vi "Grabber State Machine.vi"(8 "location of arms":dbl, 9 "grabber control buttons":T1, 10 "Limit Switches":cluster{"guideL":bool, "guideR":bool}, 11 "Laststate":T3) -> (0 "suctioncup":T2, 1 "Pickup Motor":dbl(knob) scale=-1.0..1.0, 3 "Next state":T3)   [LabVIEW 2012]
uses:
  Grabber States.ctl
  <vilib>/Rock Robotics/WPI/Solenoid/WPI_SolenoidValue.ctl
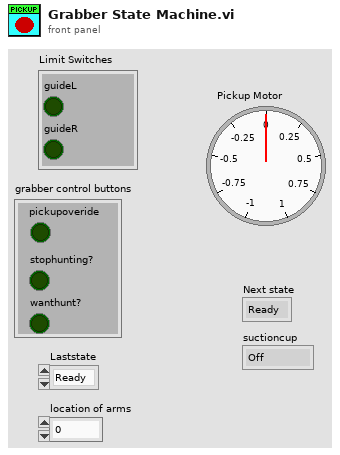
[diagram p1: front panel]
types:
  T1 = cluster{"pickupoveride":bool, "stophunting?":bool, "wanthunt?":bool}
  T2 = typedef "WPI_SolenoidValue.ctl" = enum16{"Off", "On", "Forward", "Reverse"}
  T3 = typedef "Grabber States.ctl" = enum16{"Ready", "Hunting", "Down", "Dropfrisbee"}
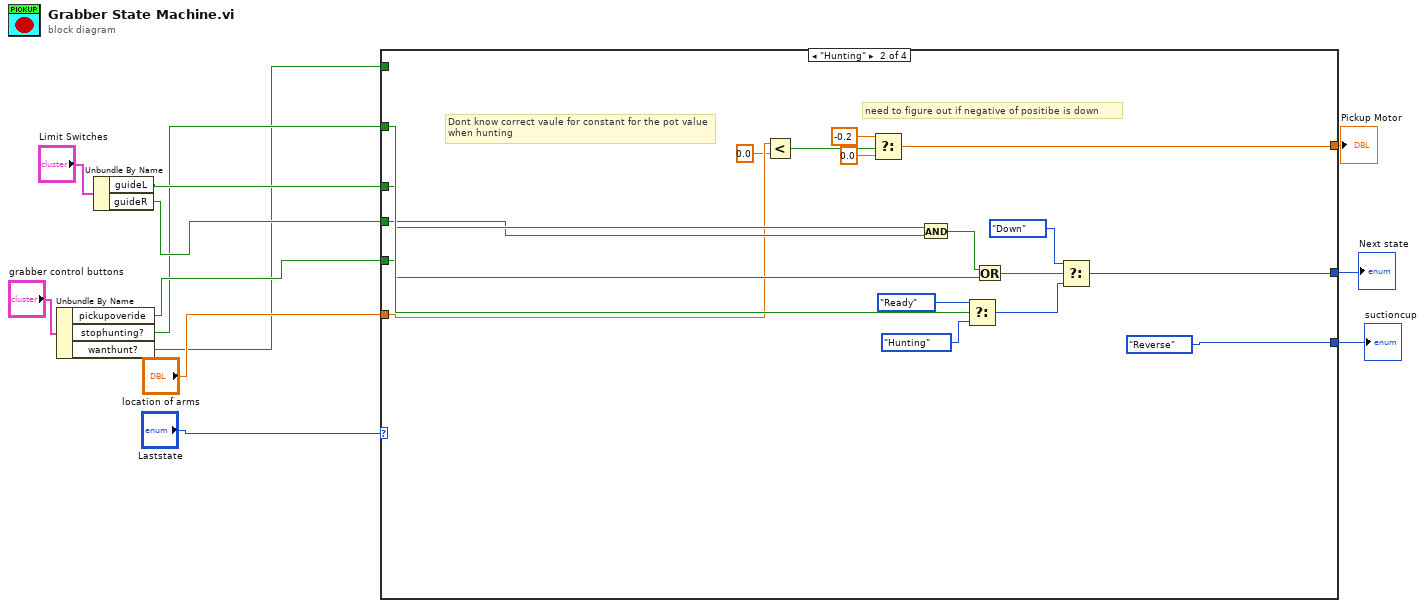
[diagram p0: block diagram]
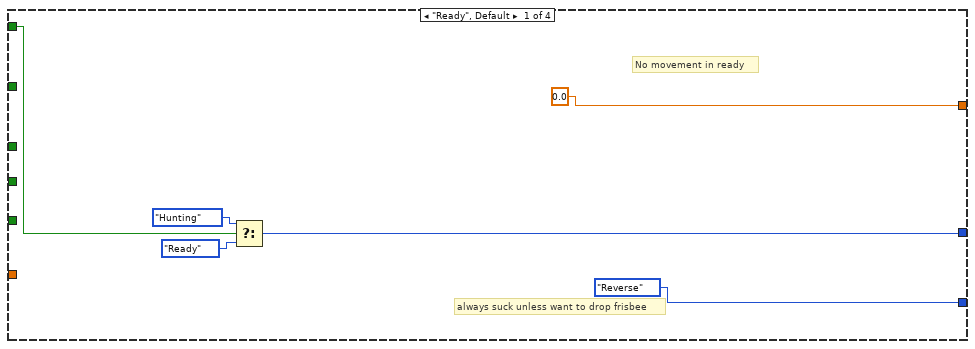
[diagram p2: hidden frame]
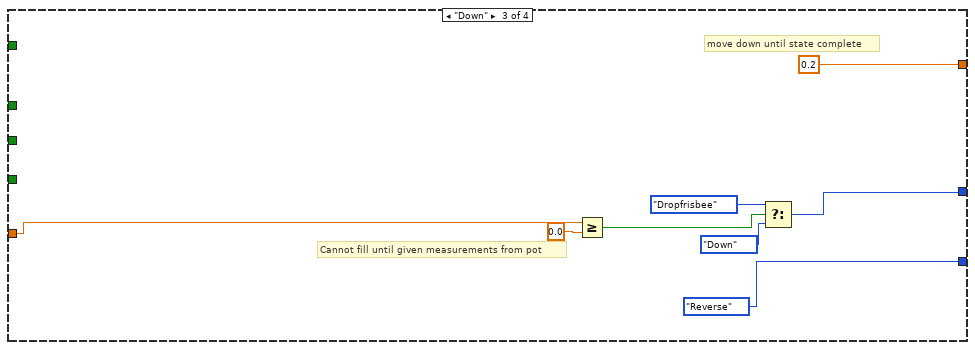
[diagram p3: hidden frame]
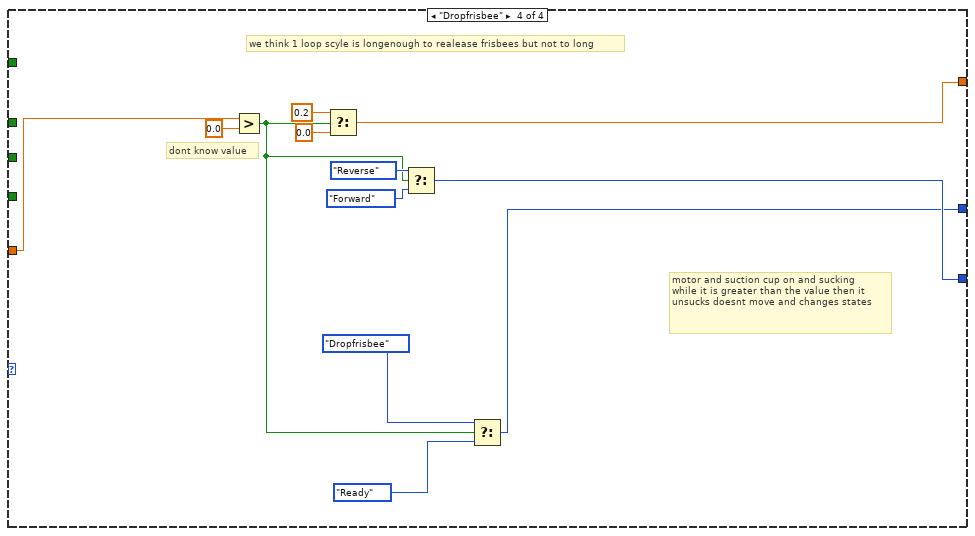
[diagram p4: hidden frame]
diagram:
  n1 = Unbundle By Name("grabber control buttons") -> ("pickupoveride"=w3:bool, "stophunting?"=w2:bool, "wanthunt?"=w1:bool)
  n2 = Unbundle By Name("Limit Switches") -> ("guideL"=w6:bool, "guideR"=w5:bool)
  n3 = case shown="\"Hunting\"" "Laststate" {
    tunnel: w1 -> [w18 _ _ _]
    tunnel: [w15 w36 w42 w46] -> w11
    tunnel: w2 -> [_ w34 _ _]
    tunnel: w6 -> [_ w30 _ _]
    tunnel: w5 -> [_ w29 _ _]
    tunnel: w3 -> [_ w27 _ _]
    tunnel: "location of arms" -> [_ w24 w40 w54]
    tunnel: [0.0 ("Pickup Motor") w19 0.2 ("f") w52] -> w9
    tunnel: [WPI_SolenoidValue."Reverse" ("suctioncup 2") WPI_SolenoidValue."Reverse" ("suctioncup 2") WPI_SolenoidValue."Reverse" ("suctioncup 2") w49] -> w8
    frame "Ready", Default {
      # "always suck unless want to drop frisbee"
      # "No movement in ready"
      n4 = Select(t=Grabber_States."Hunting" ("Enum"), s=w18, f=Grabber_States."Ready" ("Enum")) -> (s? t:f=w15:T3)
    }
    frame "Hunting" {
      # "need to figure out if negative of positibe is down"
      # "Dont know correct vaule for constant for the pot value when hunting"
      n5 = Less?(x=w24, y=0.0) -> (x < y?=w22:bool)
      n6 = Select(t=-0.2, s=w22, f=0.0) -> (s? t:f=w19:dbl)
      n7 = And(x=w30, y=w29) -> (x .and. y?=w28:bool)
      n8 = Select(t=Grabber_States."Ready" ("Enum"), s=w34, f=Grabber_States."Hunting" ("Enum")) -> (s? t:f=w35:T3)
      n9 = Or(x=w28, y=w27) -> (x .or. y?=w26:bool)
      n10 = Select(t=Grabber_States."Down" ("Enum"), s=w26, f=w35) -> (s? t:f=w36:T3)
    }
    frame "Down" {
      # "move down until state complete"
      # "Cannot fill until given measurements from pot"
      n11 = Greater Or Equal?(x=w40, y=0.0) -> (x >= y?=w41:bool)
      n12 = Select(t=Grabber_States."Dropfrisbee" ("Enum"), s=w41, f=Grabber_States."Down" ("Enum")) -> (s? t:f=w42:T3)
    }
    frame "Dropfrisbee" {
      # "motor and suction cup on and sucking\nwhile it is greater than the value then it \nunsucks doesnt move and changes states"
      # "dont know value"
      # "we think 1 loop scyle is longenough to realease frisbees but not to long"
      n13 = Greater?(x=w54, y=0.0) -> (0:w45:bool)
      n14 = Select(t=0.2, s=w45, f=0.0) -> (s? t:f=w52:dbl)
      n15 = Select(t=WPI_SolenoidValue."Reverse" ("suctioncup 2"), s=w45, f=WPI_SolenoidValue."Forward" ("suctioncup 4")) -> (s? t:f=w49:T2)
      n16 = Select(t=Grabber_States."Dropfrisbee" ("Enum"), s=w45, f=Grabber_States."Ready" ("Enum")) -> (s? t:f=w46:T3)
    }
  }
  "Pickup Motor" <- w9
  "Next state" <- w11
  "suctioncup" <- w8
